vi "Set Value (Integer).vi"(8 "error in (no error)":errorcluster, 9 "Value":i64, 10 "Feature":string, 11 "Camera in":refnum<class "Camera.lvclass">) -> (0 "error out":errorcluster, 3 "Camera":refnum<class "Camera.lvclass">)   [LabVIEW 2020, in "Camera.lvclass"]
uses:
  Camera.lvclass
  Camera.lvclass/Camera.ctl
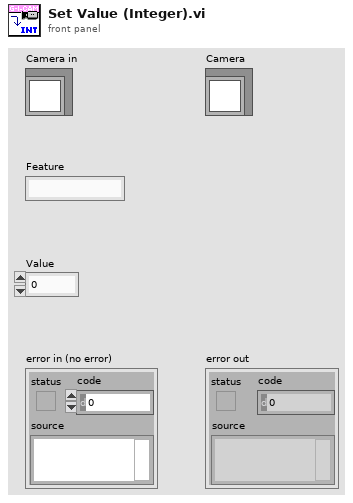
[diagram p1: front panel]
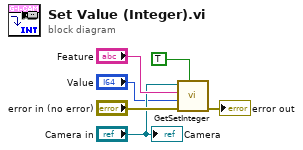
[diagram p0: block diagram]
diagram:
  n1 = call "GetSetInteger.vi"("Set?"=TRUE, "error in (no error)"="error in (no error)", "Value in"="Value", "Name"="Feature", "Camera in"="Camera in") -> ("error out"=→"error out":errorcluster)  [unwired: 5 in, 1 out]
  "Camera" <- "Camera in"
